vi "Dresser DXD Utility Clean Up Initialize.vi"(0 "VISA session":refnum<visa-resource-name>, 11 "Error In (no error)":errorcluster) -> (4 "dup VISA session":refnum<visa-resource-name>, 15 "Error Out":errorcluster)   [LabVIEW 2015]
doc: "This Utility VI closes any open VISA sessions in the event that there is an error during an initialization. It is called only from the Dresser DXD Initialize VI, and is not meant to be altered. Changing this VI can cause the Dresser DXD Initialize VI to operate improperly.\n\nWritten by:\nBLOOMY CONTROLS, INC\nWINDSOR, CT 06095, USA\n860-298-9925\nwww.bloomy.com\nV2.0.0\nMay, 2002"
panel:
  in  "VISA session (for class)":refnum<visa-resource-name>
  # "For instructions on the use of this VI, press Ctrl+H to display the help window and move the mouse over the icon, controls, and indicators"
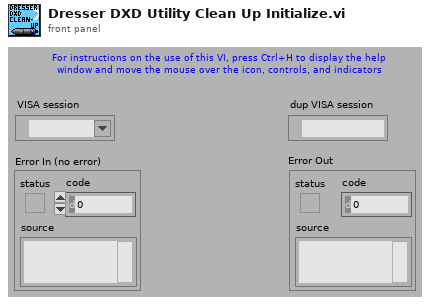
[diagram p1: front panel]
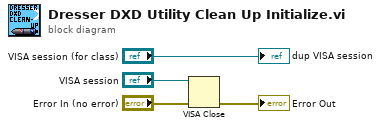
[diagram p0: block diagram]
diagram:
  n1 = VISA Close(VISA resource name="VISA session", error in (no error)="Error In (no error)") -> (error out=→"Error Out":errorcluster)
  "dup VISA session" <- "VISA session (for class)"
